vi "svinit.vi"(9 "ip":string, 11 "host?":bool) -> ()   [LabVIEW 2025]
uses:
  multi.ctl
  controls/playerstatus.ctl
  gbv.vi
panel:
  out "error out":errorcluster
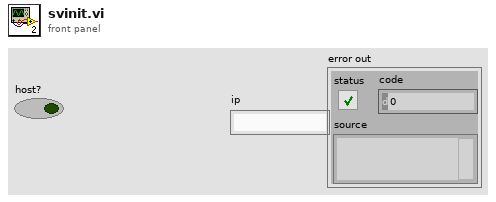
[diagram p1: front panel]
types:
  T1 = typedef "multi.ctl" = cluster{"Array":i8[][][], "player":T2[], "layer":i32, "size":i32, "mode":u16, "sec":i32, "minecount":i32}
  T2 = typedef "playerstatus.ctl" = cluster{"correct flag":i32, "wrong flag":i32, "username":string, "status":u16}
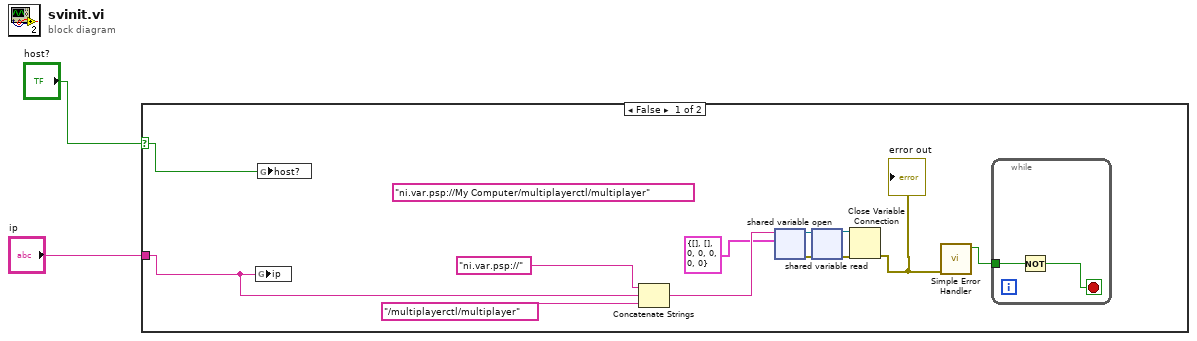
[diagram p0: block diagram]
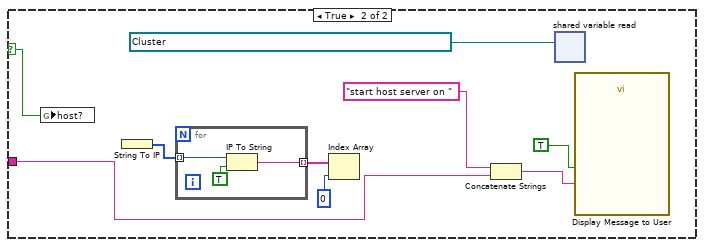
[diagram p2: hidden frame]
diagram:
  n1 = case shown="False" "host?" {
    selector: "host?" -> [w14 w25]
    tunnel: "ip" -> [w13 w17]
    frame False {
      (unwired) "ni.var.psp://My Computer/multiplayerctl/multiplayer"
      n2 = global write "gbv.vi" "ip"(w13) -> ()
      n3 = global write "gbv.vi" "host?"(w14) -> ()
      n4 = Concatenate Strings("ni.var.psp://" ("string"), w13, "/multiplayerctl/multiplayer" ("string")) -> (w9:string)
      n5 = shared-variable-open(w9, T1 {"Array"=[], "player"=[], "layer"=0, "size"=0, "mode"=0, "sec"=0, "minecount"=0} ("data out")) -> (w7:refnum<k21>, w6:errorcluster)  [unwired: 2 in]
      n6 = shared-variable-read(w7, w6) -> (w5:refnum<k21>, w4:errorcluster)  [unwired: 2 out]
      n7 = Close Variable Connection(8:w4, 11:w5) -> (0:w3:errorcluster)
      "error out" <- w3
      n8 = call <vilib>:"Simple Error Handler.vi"("error in (no error)"=w3) -> ("error?"=w10:bool)  [unwired: 4 in, 4 out]
      n9 = while {
        tunnel: w10 -> [w16]
        stop <- w15 stop-if-true
        n10 = Not(x=w16) -> (.not. x?=w15:bool)
      }
    }
    frame True {
      n11 = global write "gbv.vi" "host?"(w25) -> ()
      n12 = String To IP() -> (0:w22:u32[])  [unwired: 1 in]
      n13 = for {
        tunnel: w22 -> [w28] mode=indexing
        tunnel: [w27] -> w23 mode=indexing
        n14 = IP To String(1:TRUE ("dot notation? (F)"), 2:w28) -> (0:w27:string)
      }
      n15 = Index Array(array=w23, index=0) -> ()  [unwired: 1 out]
      n16 = Concatenate Strings("start host server on " ("string"), w17) -> (w24:string)
      n17 = shared-variable-read(refnum<k21> "ni.var.psp://My Computer/multiplayerctl/multiplayer" ("shared variable refnum in")) -> ()  [unwired: 1 in, 3 out]
      n18 = call "Display Message to User"("Enable"=TRUE, "Message"=w24) -> ()  [unwired: 8 in, 2 out]
    }
  }
